vi "FPGA_target_command_handler.vi"(0 "mem_addr_in":u32, 1 "mem_addr_start":u32, 3 "force_stop":bool, 4 "stop_execution_in":bool, 5 "FIFO_full":bool, 6 "continuous":bool, 7 "mem_data_in":T1) -> (10 "mem2_addr":u32, 11 "start_sctl":bool, 12 "mem2_data":u32, 13 "mem_data_out":T1, 14 "mem_addr_ out":u32, 17 "stop_execution_out":bool, 18 "stop_triggered":bool, 19 "write_FIFO":bool)   [LabVIEW 2014]
doc: "Reads data from the internal memory of the FPGA and provides output that will be used later-on to be filled into an internal FIFO"
uses:
  FPGA_mem_data_type.ctl
panel:
  # "<-- renamed"
  # "<-- renamed"
  # "--> new control/ indicator which are connected to new shift-register <--"
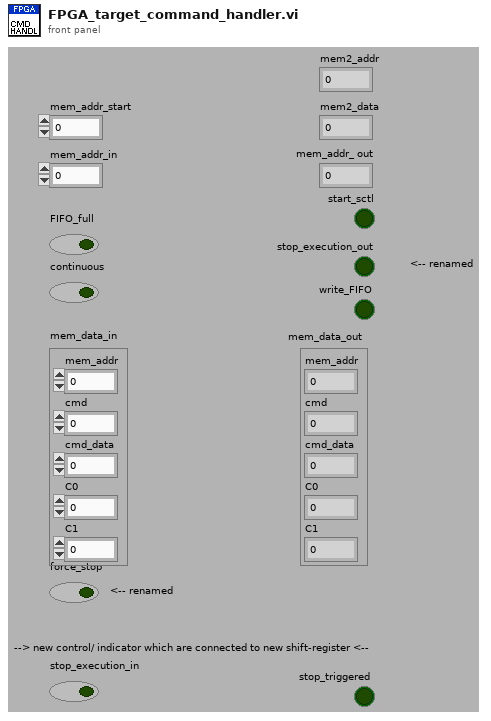
[diagram p1: front panel]
types:
  T1 = typedef "FPGA_mem_data_type.ctl" = cluster{"mem_addr":u32, "cmd":u8, "cmd_data":u32, "C0":u32, "C1":u32}
  T2 = cluster{"addr_dup":u32, "Mem 0 data":u8, "data_mem3":u32, "data_mem1":u32, "data_mem2":u32}
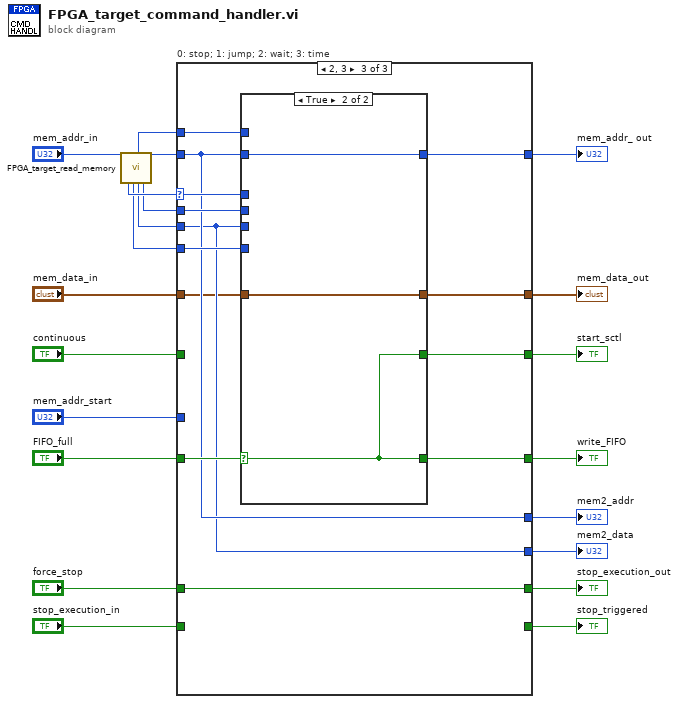
[diagram p0: block diagram]
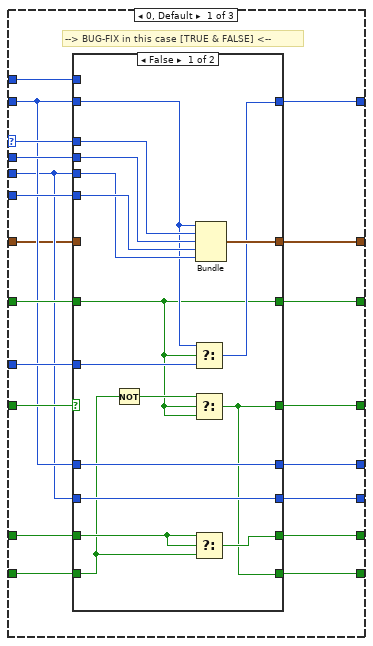
[diagram p2: hidden frame]
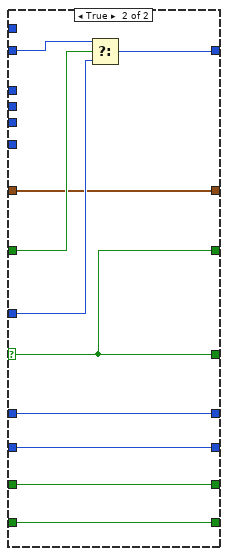
[diagram p3: hidden frame]
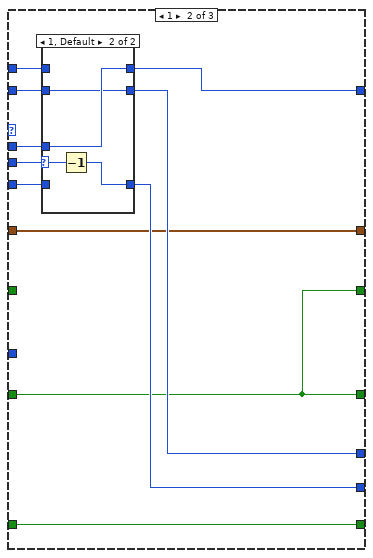
[diagram p4: hidden frame]
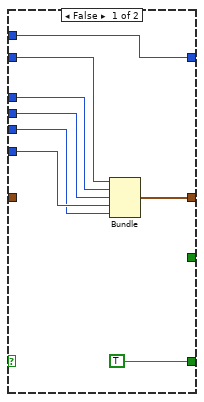
[diagram p6: hidden frame]
diagram:
  n1 = call "FPGA_target_read_memory.vi"("addr_in"="mem_addr_in") -> ("data_mem0"=w13:u8, "data_mem1"=w9:u32, "next_addr_out"=w8:u32, "data_mem2"=w10:u32, "data_mem3"=w11:u32, "addr_dup"=w12:u32)  [unwired: 13 in]
  n2 = case "0: stop; 1: jump; 2: wait; 3: time" shown="2, 3" w13 {
    selector: w13 -> [w36 _ w95]
    tunnel: w12 -> [w28 w78 w89]
    tunnel: [w40 w73 w91] -> w5
    tunnel: w10 -> [w26 w75 w88]
    tunnel: [w38 w68 w90] -> w21
    tunnel: [w39 w68 w96] -> w19
    tunnel: w11 -> [w35 w77 w94]
    tunnel: "continuous" -> [w33 _ _]
    tunnel: "mem_addr_start" -> [w32 _ _]
    tunnel: w9 -> [w34 w76 w93]
    tunnel: "FIFO_full" -> [w41 w68 w97]
    tunnel: w8 -> [w37 w74 w92]
    tunnel: "force_stop" -> [w31 w72 w98]
    tunnel: [w30 w72 w98] -> w14
    tunnel: [w29 w71 w89] -> w7
    tunnel: [w27 w70 w88] -> w6
    tunnel: [w24 w69 w87] -> w4
    tunnel: "mem_data_in" -> [w25 w69 w86]
    tunnel: "stop_execution_in" -> [w23 _ _]
    tunnel: [w22 _ _] -> w1
    frame 0, Default {
      # "--> BUG-FIX in this case [TRUE & FALSE] <--"
      n3 = case shown="False" w41 {
        selector: w41 -> [_ w67]
        tunnel: w28 -> [w49 w60]
        tunnel: [w47 w63] -> w40
        tunnel: [w43 w67] -> w39
        tunnel: [w42 w67] -> w38
        tunnel: w37 -> [_ _]
        tunnel: w36 -> [w53 _]
        tunnel: w35 -> [w52 _]
        tunnel: w34 -> [w51 _]
        tunnel: w26 -> [w50 _]
        tunnel: w33 -> [w42 w62]
        tunnel: w32 -> [w48 w61]
        tunnel: w31 -> [w57 w66]
        tunnel: [w44 w66] -> w30
        tunnel: w28 -> [w56 w65]
        tunnel: [w56 w65] -> w29
        tunnel: w26 -> [w55 w64]
        tunnel: [w55 w64] -> w27
        tunnel: w25 -> [_ w59]
        tunnel: [w54 w59] -> w24
        tunnel: w23 -> [w45 w58]
        tunnel: [w43 w58] -> w22
        frame False {
          n4 = Not(x=w45) -> (.not. x?=w46:bool)
          n5 = Select(t=w49, s=w42, f=w48) -> (s? t:f=w47:u32)
          n6 = Select(t=w46, s=w42, f=w42) -> (s? t:f=w43:bool)
          n7 = Select(t=w57, s=w57, f=w45) -> (s? t:f=w44:bool)
          n8 = Bundle("addr_dup"=w49, "Mem 0 data"=w53, "data_mem3"=w52, "data_mem1"=w51, "data_mem2"=w50) -> (w54:T2)  [unwired: 1 in]
        }
        frame True {
          n9 = Select(t=w60, s=w62, f=w61) -> (s? t:f=w63:u32)
        }
      }
    }
    frame 1 {
      n10 = case shown="1, Default" w75 {
        selector: w75 -> [_ w84]
        tunnel: [w81 w85] -> w73
        tunnel: w78 -> [w80 w83]
        tunnel: w77 -> [_ w85]
        tunnel: w76 -> [w79 _]
        tunnel: w74 -> [w81 _]
        tunnel: [w80 w83] -> w71
        tunnel: [w79 w82] -> w70
        frame 0 {
        }
        frame 1, Default {
          n11 = Decrement(x=w84) -> (x-1=w82:u32)
        }
      }
    }
    frame 2, 3 {
      n12 = case shown="True" w97 {
        selector: w97 -> [_ w109]
        tunnel: [TRUE w109] -> w96
        tunnel: w95 -> [w103 _]
        tunnel: w94 -> [w102 _]
        tunnel: w93 -> [w101 _]
        tunnel: w88 -> [w100 _]
        tunnel: w92 -> [w106 _]
        tunnel: [w106 w108] -> w91
        tunnel: w89 -> [w104 w108]
        tunnel: [_ w109] -> w90
        tunnel: [w99 w107] -> w87
        tunnel: w86 -> [_ w107]
        frame False {
          n13 = Bundle("addr_dup"=w104, "Mem 0 data"=w103, "data_mem3"=w102, "data_mem1"=w101, "data_mem2"=w100) -> (w99:T2)  [unwired: 1 in]
        }
        frame True {
        }
      }
    }
  }
  "mem_addr_ out" <- w5
  "start_sctl" <- w21
  "write_FIFO" <- w19
  "stop_execution_out" <- w14
  "mem2_addr" <- w7
  "mem2_data" <- w6
  "mem_data_out" <- w4
  "stop_triggered" <- w1
